vi "SoundMeasureWunan.vi"() -> ()   [LabVIEW 2016]
uses:
  <vilib>/Instr/_visa.llb/VISA Configure Serial Port (Instr).vi
  <vilib>/Utility/config.llb/Read Key (Double).vi
  <vilib>/Utility/file.llb/Write Delimited Spreadsheet (DBL).vi
  <vilib>/Utility/config.llb/NI_LVConfig.lvlib
panel:
  in  "record cycle":u64=7 min=6 step=1
  in  "freq (MHz)":dbl=1.36 min=0.1 max=10.0 step=0.01
  in  "SETVOLT":bool
  out "error out":errorcluster
  in  "cycle":u32=120
  in  "Channel":u16
  in  "KYCT axis in HIFU coordinate":cluster{"X axis":dbl[], "Z axis":dbl[]}={"X axis"=[1.0, 0.0, 0.0], "Z axis"=[0.0, 0.0, 1.0]}
  in  "KYCT coordinate":T1
  in  "Sens (V/MPa)":dbl=0.1284
  in  "Port":u32=12321
  in  "HIFU_connect":bool
  in  "HIFU_Telnet":bool
  out "Pressure (MPa)":dbl format="%#_4g"
  in  "pout":bool
  in  "totle chnnum":i16=64
  in  "HIFU IP":string="192.168.1.72"
  in  "SETPHS":bool
  out "XY Graph 2":T2(graph)
  in  "Set global voltage":bool
  in  "Voltage":dbl=4.0 min=0.5 max=20.0 step=1.0
  out "Sonication":bool
  in  "continuousOut":bool
  in  "Scan":bool
  in  "Tab Control":enum32{"1D Scan", "2D Scan", "Monitor"}(tab)
  out "1D plot":cluster{dbl[], dbl[]}(graph)
  out "2D Scan":dbl[][](graph)
  in  "start":bool
  in  "reord":bool
  out "Current":dbl[](graph)
  out "Voltage":dbl[](graph)
  in  "Go":bool
  in  "Speed":dbl=0.5 min=0.2 max=2.5 step=0.1
  in  "Position":dbl[](array[numeric]) step=5.0 format="%#_6f"
  in  "Z+":bool
  in  "Z-":bool
  in  "Y+":bool
  in  "Y-":bool
  in  "X+":bool
  in  "X-":bool
  in  "error in (no error)":errorcluster
  out "HIFU":bool
  out "osc":bool
  out "KYCT":bool
  in  "Exit":bool
  in  "3D motorized stage":refnum<visa-resource-name>
  in  "oscilloscope":refnum<visa-resource-name>
  # "Z"
  # "X"
  # "Y"
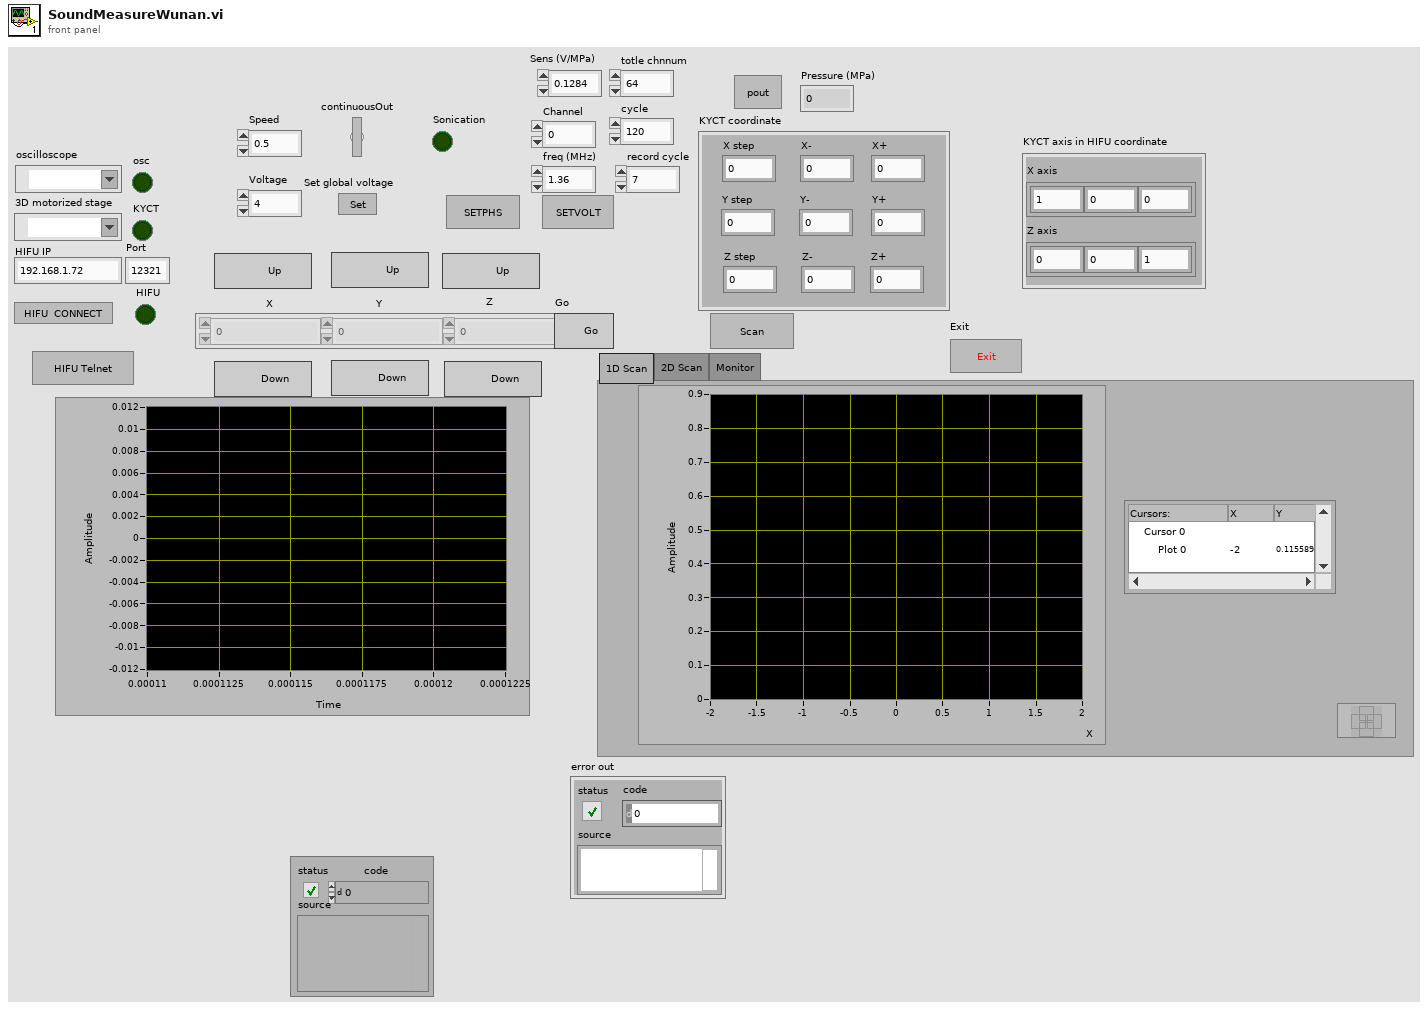
[diagram p1: front panel]
types:
  T1 = cluster{"X-":dbl, "X step":dbl, "Y-":dbl, "Y step":dbl, "Z-":dbl, "Z step":dbl, "Z+":dbl, "X+":dbl, "Y+":dbl}
  T2 = cluster{"time sequence":dbl[], "Voltage sequence":dbl[]}
  T3 = enum8{"Enabled", "Disabled", "Disabled and Grayed Out"}
  T4 = typedef "NI_LVConfig.lvlib/Config Data RefNum.ctl" = refnum<k1>
  T5 = typedef "NI_Matrix.lvlib/RealMatrix.ctl" = dbl[][]
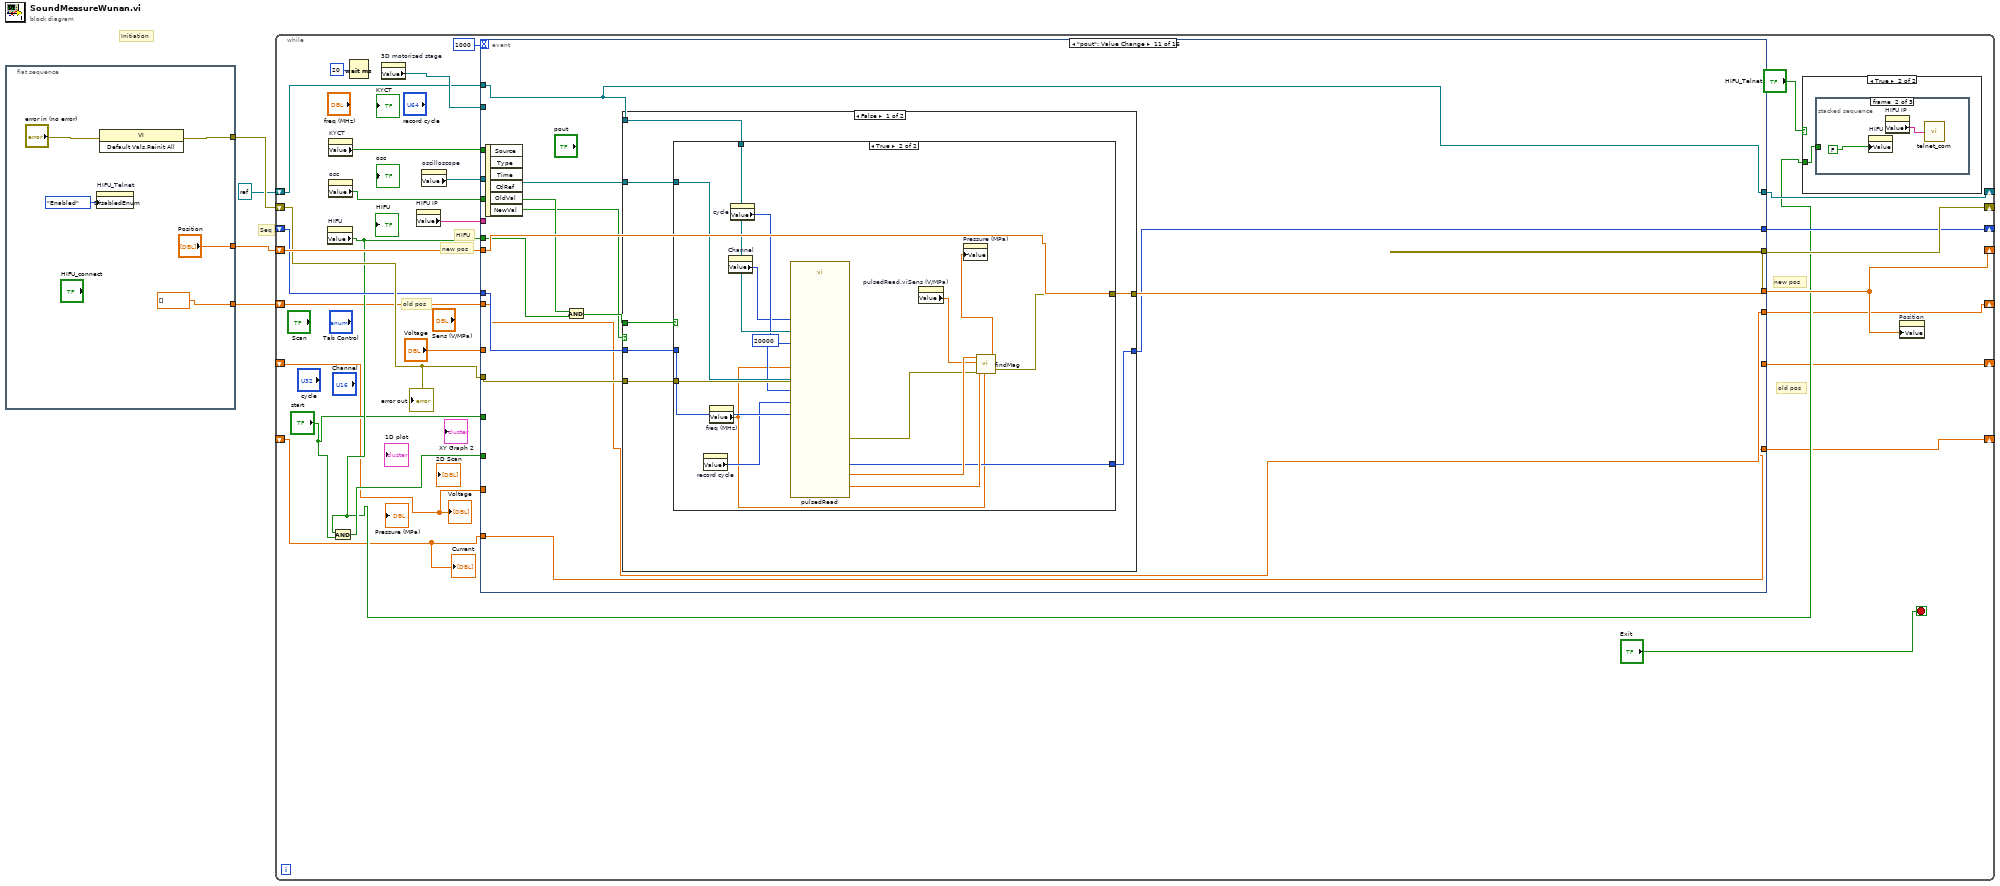
[diagram p0: block diagram]
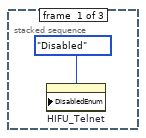
[diagram p3: hidden frame]
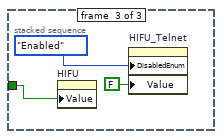
[diagram p4: hidden frame]
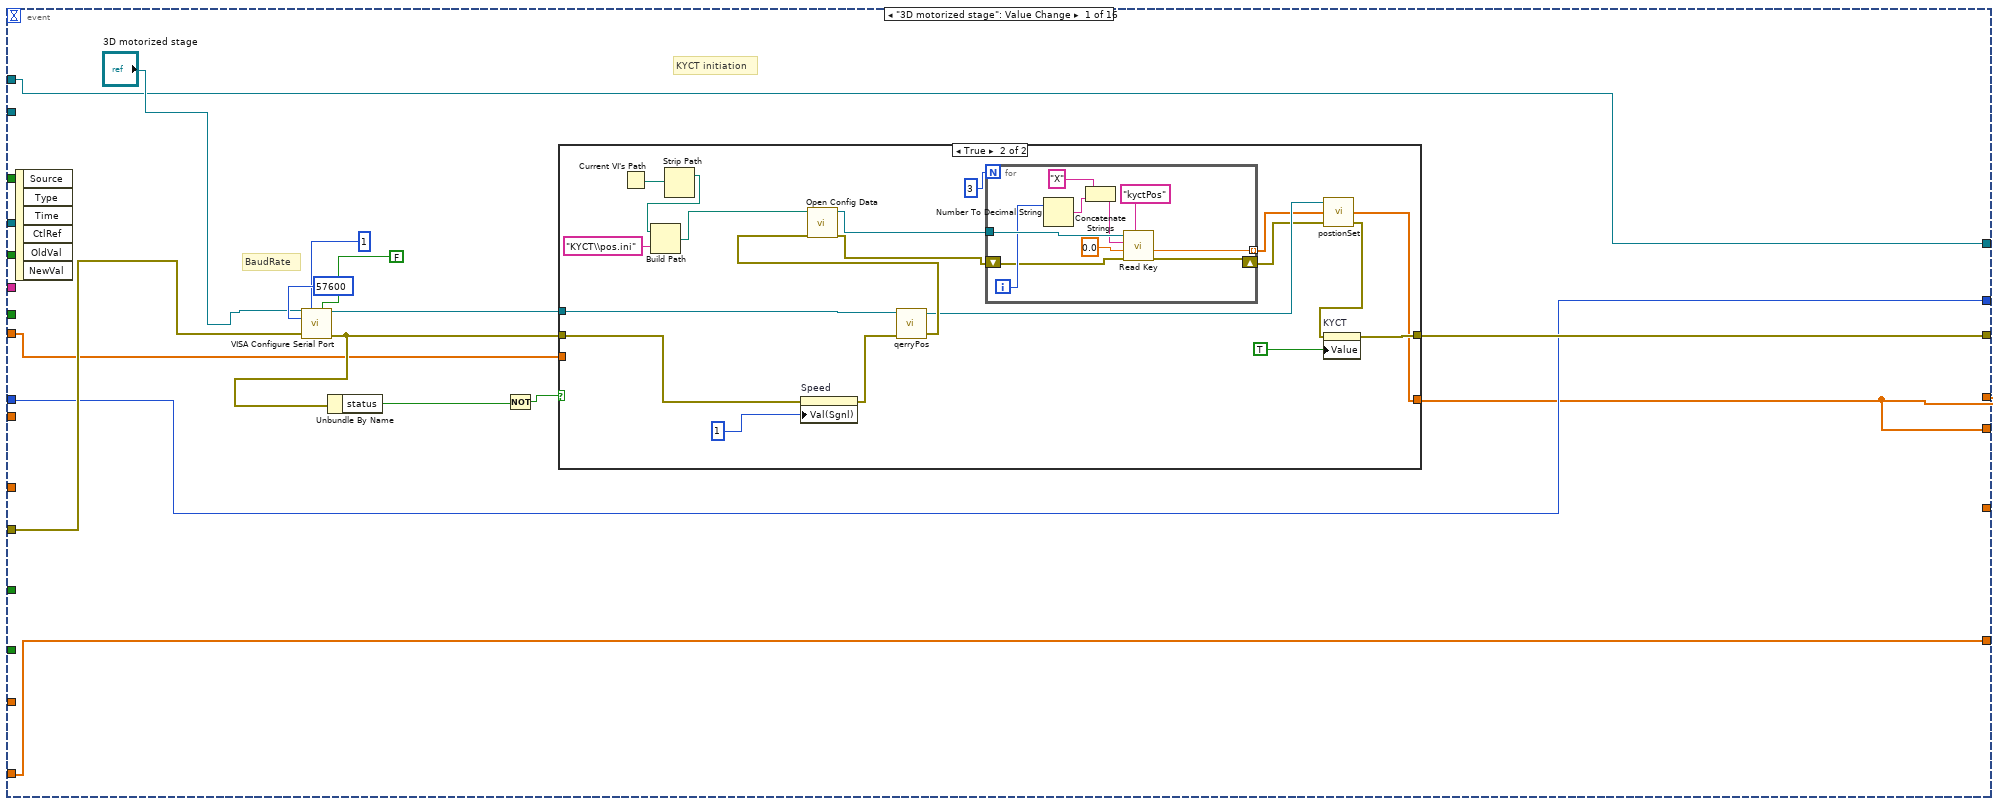
[diagram p5: hidden frame]
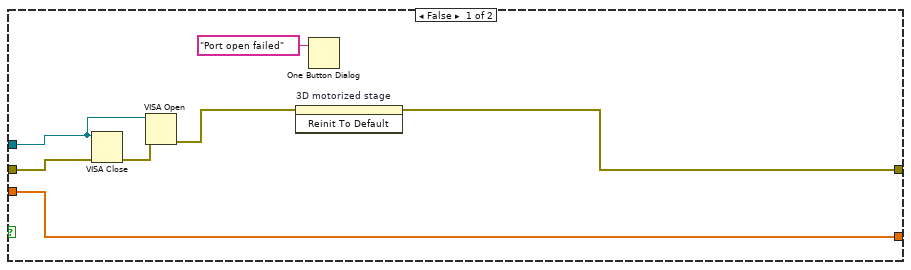
[diagram p6: hidden frame]
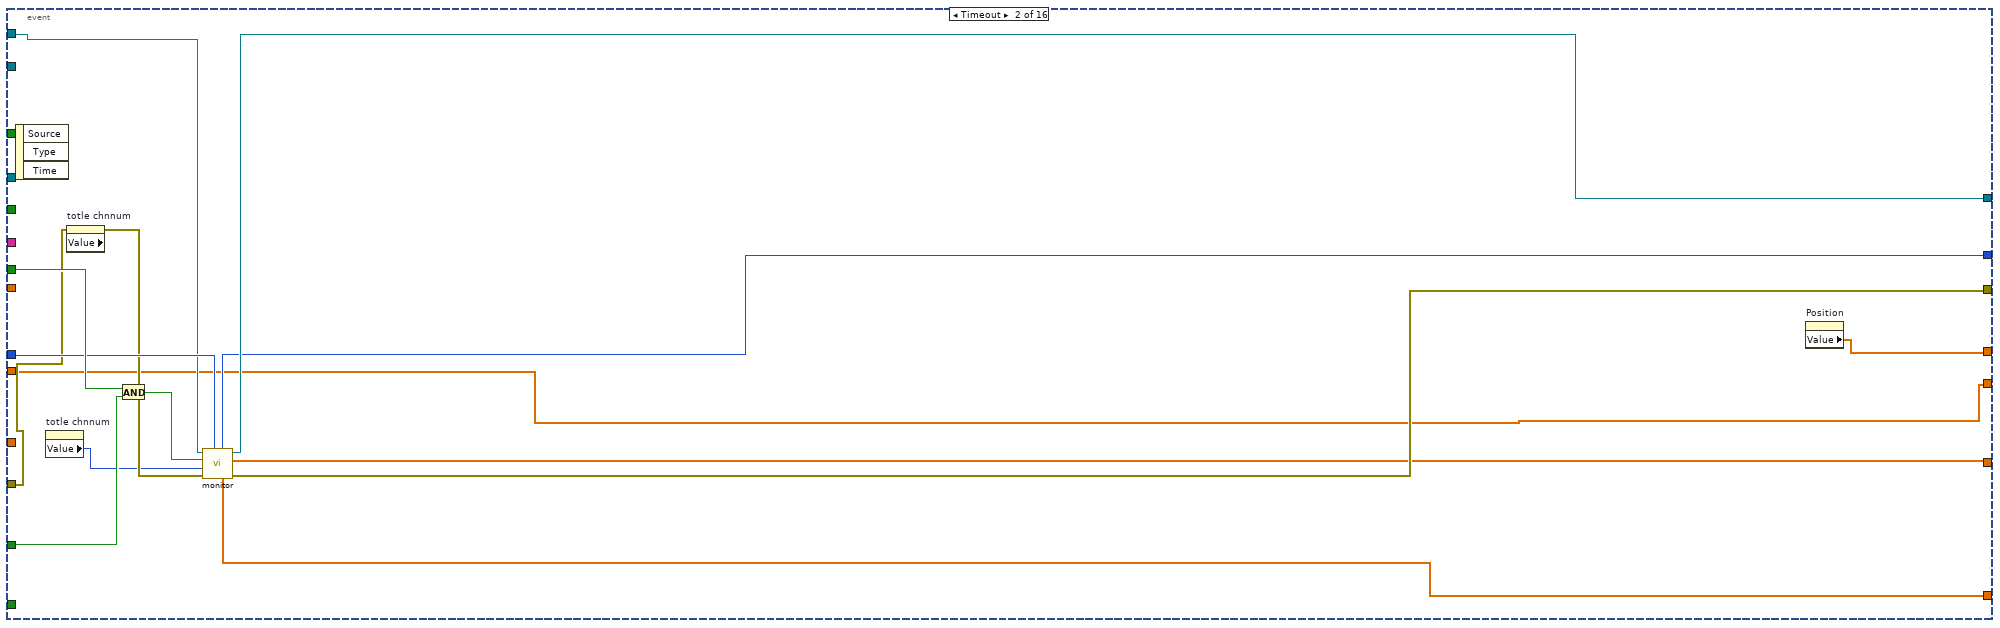
[diagram p7: hidden frame]
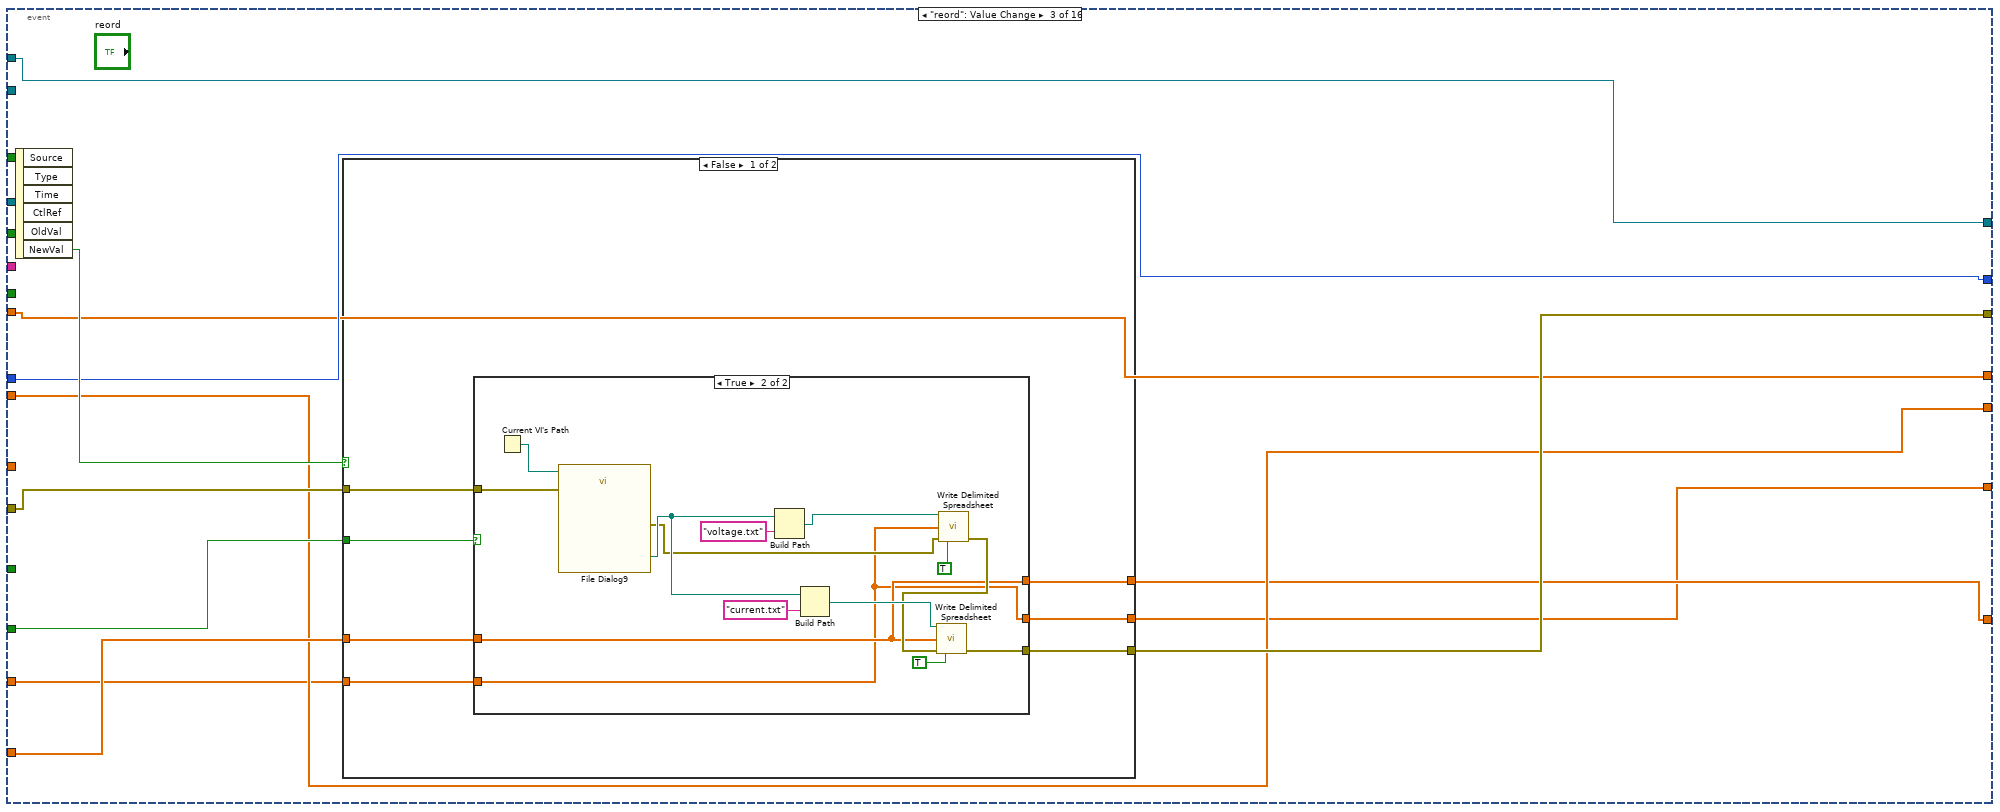
[diagram p8: hidden frame]
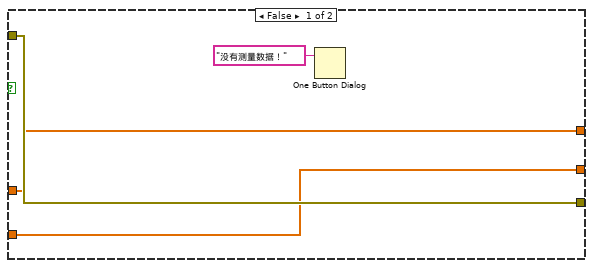
[diagram p9: hidden frame]
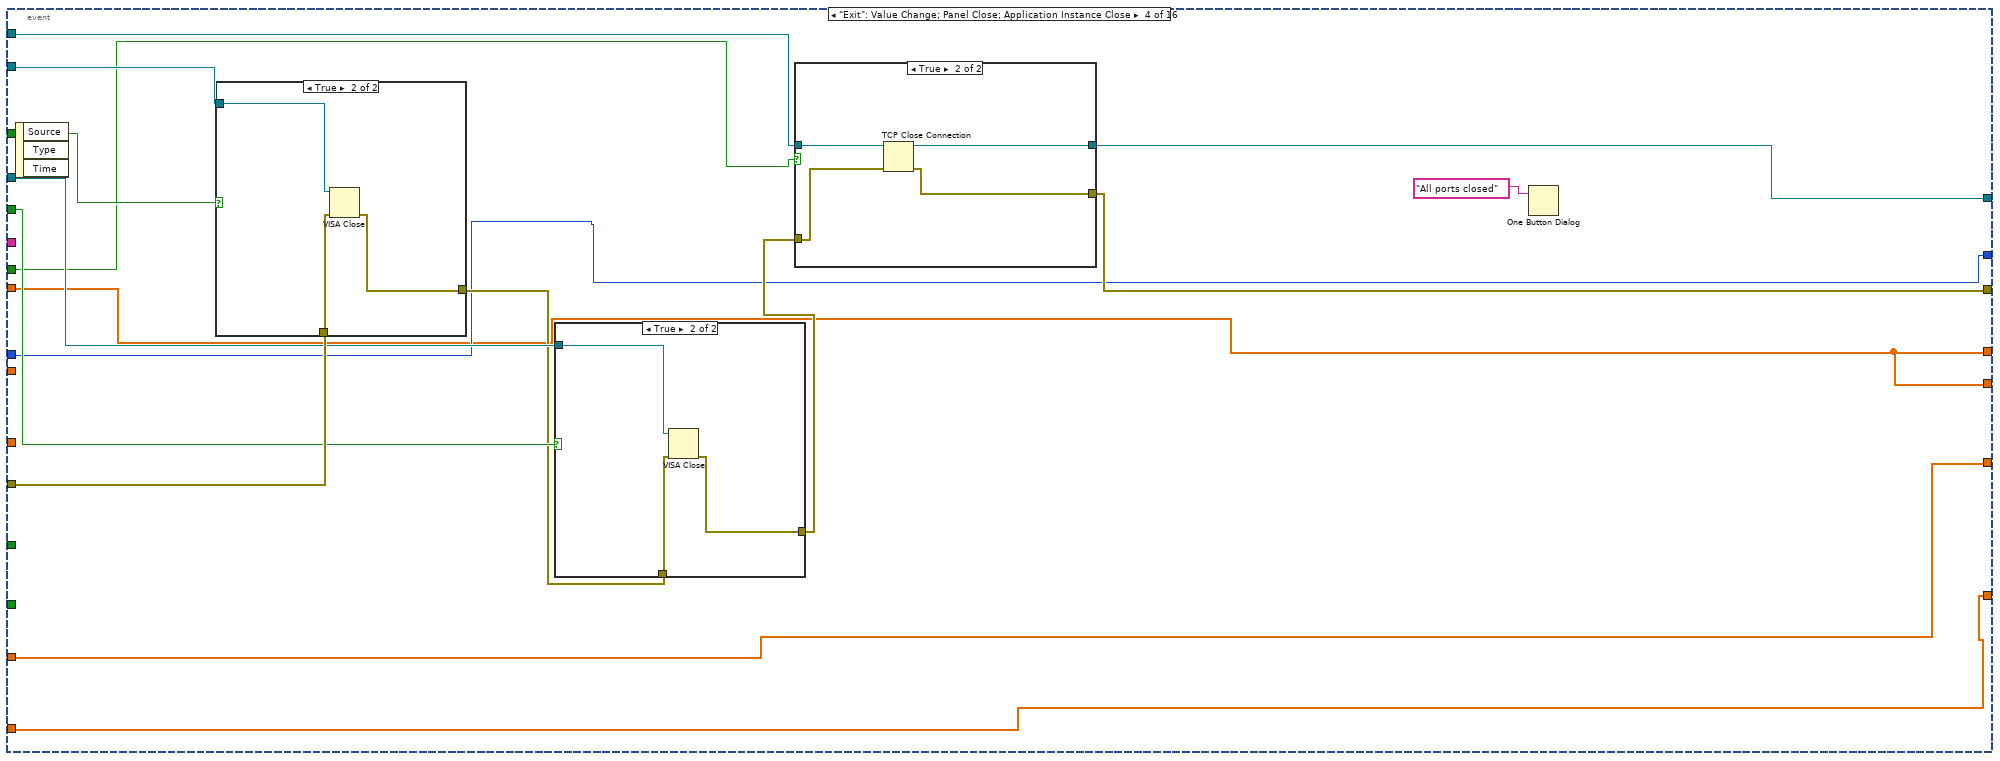
[diagram p11: hidden frame]
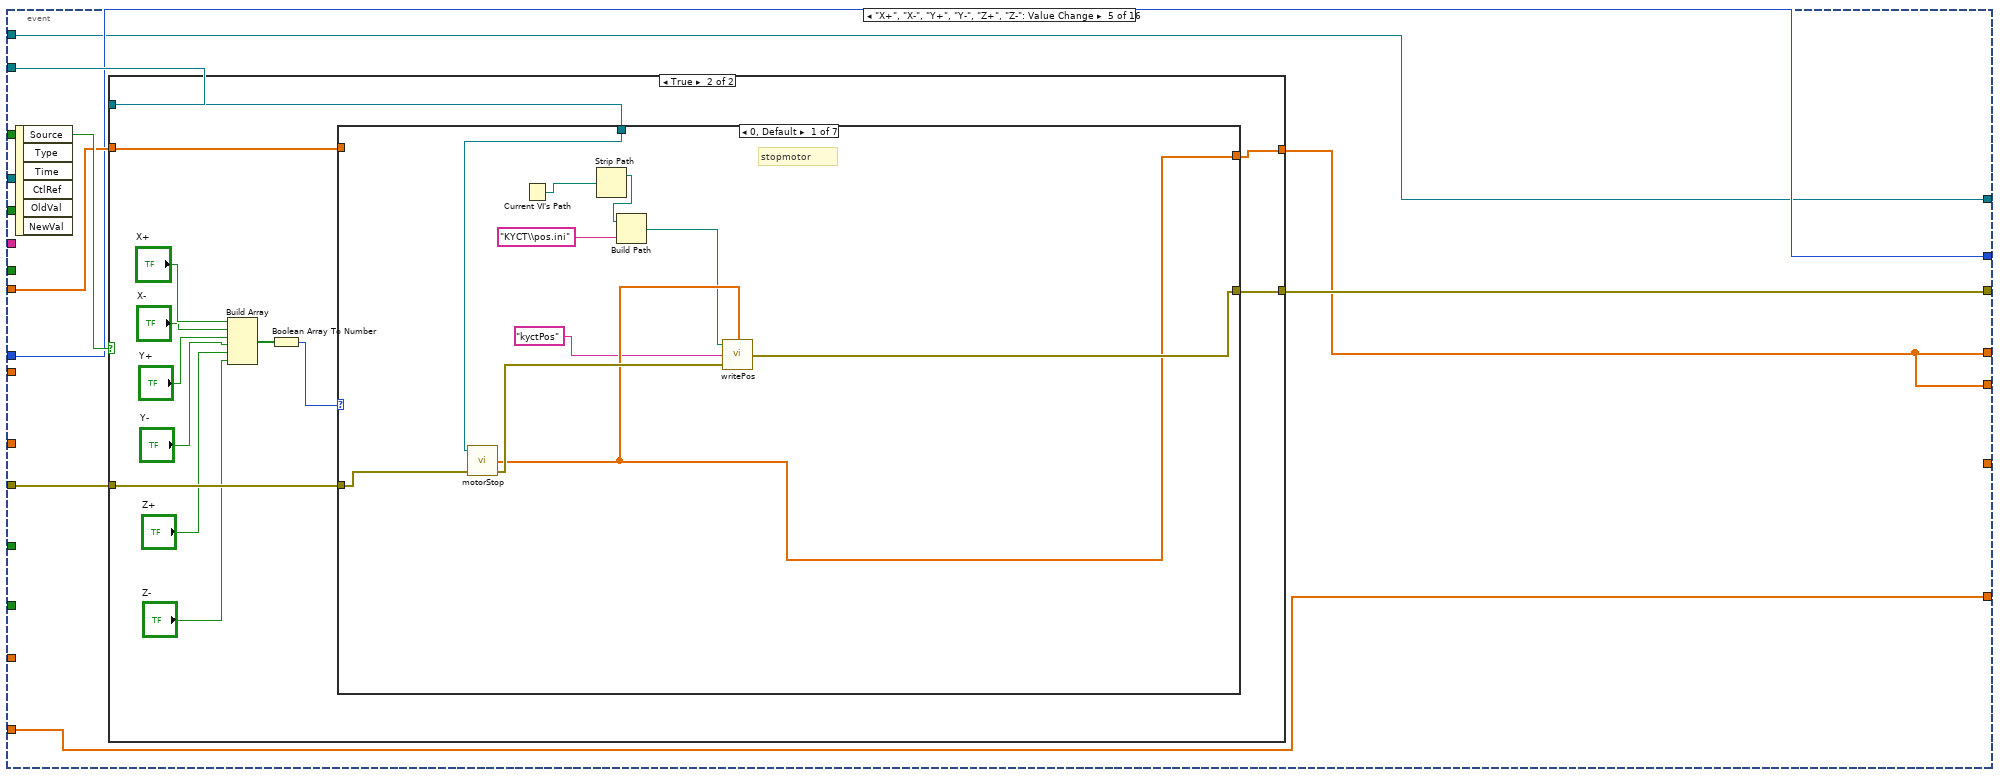
[diagram p15: hidden frame]
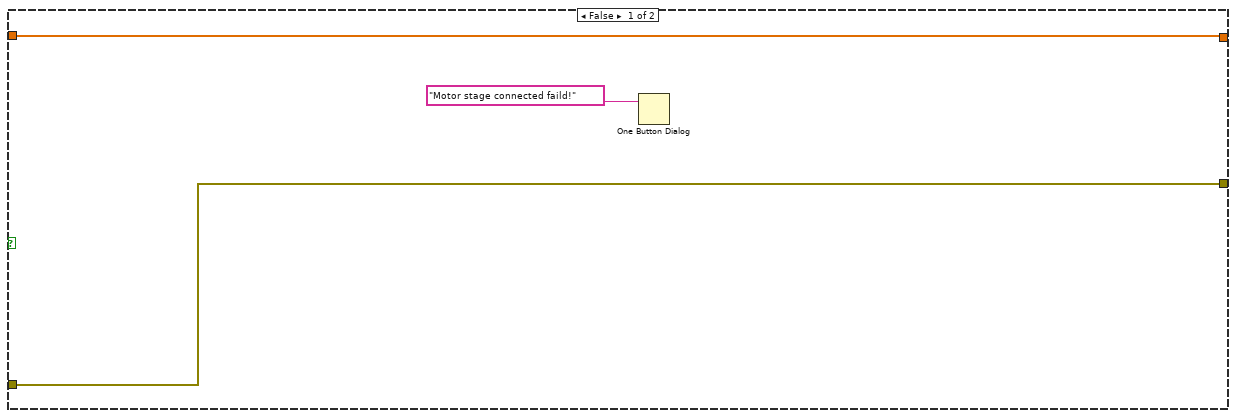
[diagram p16: hidden frame]
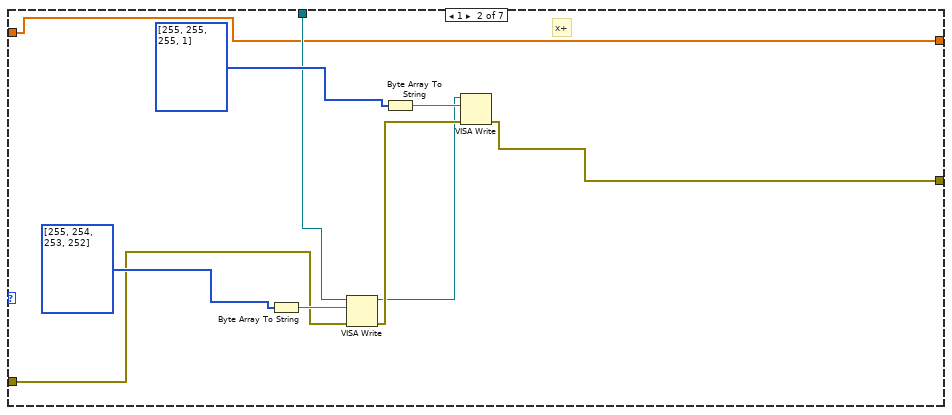
[diagram p17: hidden frame]
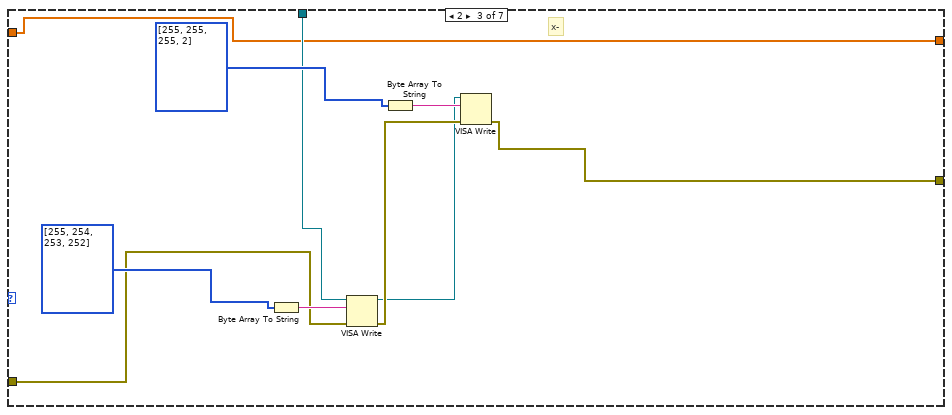
[diagram p18: hidden frame]
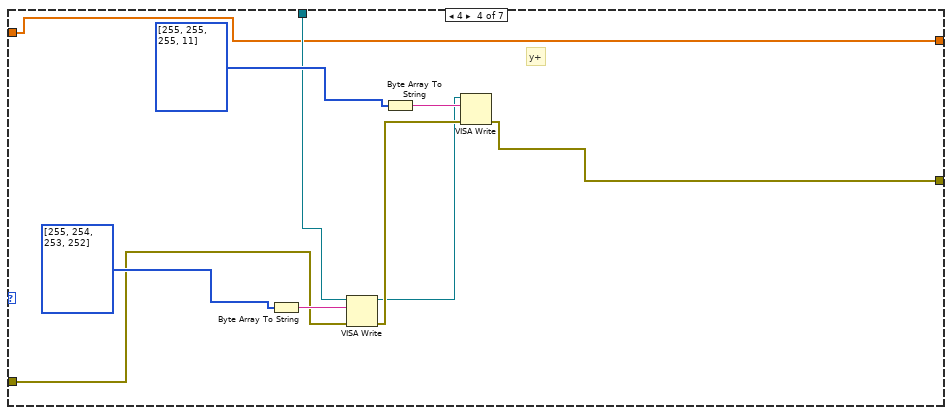
[diagram p19: hidden frame]
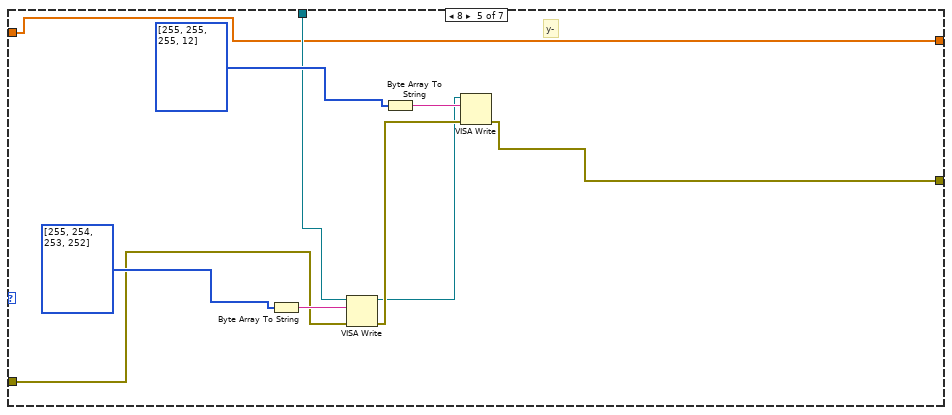
[diagram p20: hidden frame]
diagram:
  # "Seq"
  # "Initiation"
  n1 = flat-sequence {
    tunnel: ["Position"] -> w4
    tunnel: [w8] -> w3
    tunnel: [dbl[] []] -> w1
    frame #0 {
      n2 = property on="HIFU_Telnet" class="Bool (strict)"("DisabledEnum"=T3."Enabled" ("Disabled")) -> ()  [unwired: 2 in, 2 out]
      n3 = invoke class="VI" method="Default Vals.Reinit All"(error in="error in (no error)") -> (error out=w8:errorcluster)  [unwired: 2 in, 2 out]
    }
  }
  n4 = while {
    shift-right: [w34] -> _
    shift-left: w4 -> [w33]
    shift-right: [w32] -> _
    shift-left: w3 -> [w20]
    shift-right: [w23] -> _
    shift-left: refnum<k5> refnum ("connection ID out") -> [w22]
    shift-right: [w21] -> _
    shift-left: _ -> [w19]
    shift-right: [w17] -> _
    shift-left: _ -> [w16]
    shift-right: [w13] -> _
    shift-left: w1 -> [w12]
    shift-right: [w11] -> _
    shift-left: _ -> [w10]
    stop <- "Exit" stop-if-true
    # "HIFU"
    # "old pos"
    # "new pos"
    # "old pos"
    # "new pos"
    n5 = property on="HIFU" class="Bool (strict)"() -> ("Value"=w18:bool)  [unwired: 2 in, 2 out]
    n6 = property on="KYCT" class="Bool (strict)"() -> ("Value"=w36:bool)  [unwired: 2 in, 2 out]
    n7 = property on="osc" class="Bool (strict)"() -> ("Value"=w35:bool)  [unwired: 2 in, 2 out]
    n8 = And(x=w18, y="start") -> (x .and. y?=w25:bool)
    n9 = Wait (ms)(milliseconds to wait=u32 20) -> ()  [unwired: 1 out]
    n10 = property on="3D motorized stage" class="VISAName"() -> ("Value"=w30:refnum<visa-resource-name>)  [unwired: 2 in, 2 out]
    n11 = property on="HIFU IP" class="Str"() -> ("Value"=w26:string)  [unwired: 2 in, 2 out]
    n12 = property on="oscilloscope" class="VISAName"() -> ("Value"=w29:refnum<visa-resource-name>)  [unwired: 2 in, 2 out]
    n13 = event shown="[10] \"pout\": Value Change" {
      selector: _ -> [_ _ _ _ _ _ _ _ _ _ _ _ _ _ _ _]
      dyn-events: _ -> [_ _ _ _ _ _ _ _ _ _ _ _ _ _ _ _]
      timeout: 1000 -> [_ _ _ _ _ _ _ _ _ _ _ _ _ _ _ _]
      tunnel: w30 -> [_ _ _ w164 w187 w283 w304 _ _ w423 _ _ _ _ _ _]
      tunnel: w29 -> [_ _ _ w161 _ _ _ _ _ w421 w659 _ _ _ _ _]
      tunnel: w20 -> [w54 w107 w121 w163 w186 w284 w303 w335 w377 w422 w658 w699 w709 w745 w760 w792]
      tunnel: w36 -> [_ _ _ w165 w188 w282 w305 _ _ w428 _ _ _ _ _ w796]
      tunnel: [w56 w99 w119 w155 w185 w280 w301 w333 w375 w420 w657 w698 w707 w745 w759 w791] -> w32
      tunnel: w35 -> [_ _ _ w162 _ _ _ _ _ w427 w656 _ _ _ _ _]
      tunnel: w33 -> [w49 _ w114 w152 w184 w277 _ w336 w378 w419 w660 w700 w710 w747 w757 w795]
      tunnel: [w45 w97 w114 w152 w181 w277 w296 w336 w378 w413 w660 w700 w710 w747 w757 w794] -> w34
      tunnel: w18 -> [_ w109 _ w158 _ _ _ w334 w376 w426 w655 _ _ _ w756 w789]
      tunnel: "Voltage" -> [_ _ _ _ _ _ _ _ _ _ _ _ _ _ w758 _]
      tunnel: w16 -> [w44 _ w120 w150 w180 w275 w293 w327 w369 w411 w648 w693 w702 w749 w750 w782]
      tunnel: w26 -> [_ _ _ _ _ _ _ _ _ w418 _ _ _ _ _ w788]
      tunnel: w25 -> [_ _ w118 _ _ _ _ _ _ _ _ _ _ _ _ _]
      tunnel: [w47 w103 w116 w153 w182 w278 w298 w331 w373 w414 w650 w695 w705 w743 w752 w784] -> w23
      tunnel: w22 -> [w47 w104 w116 w156 w182 w278 w298 w331 w373 w414 w650 w695 _ w743 w752 w787]
      tunnel: [w46 w101 w115 w154 w183 w279 w299 w329 w371 w415 w651 w696 w704 w744 w753 w785] -> w21
      tunnel: w19 -> [w46 w108 w115 w154 w183 w279 w299 w330 w372 w416 w652 w696 _ w744 w754 w786]
      tunnel: [w44 w102 w111 w150 w180 w275 w293 w327 w369 w411 w648 w693 w702 w749 w750 w782] -> w17
      tunnel: "start" -> [_ w100 _ _ _ _ _ _ _ _ _ _ _ _ _ _]
      tunnel: [w45 w96 w113 w152 w181 w276 w295 w328 w370 w413 w649 w694 w703 w746 w751 w783] -> w13
      tunnel: w12 -> [_ w96 w113 _ _ w276 w297 w328 w370 w412 w649 w694 w703 w746 w751 w783]
      tunnel: [_ w95 w110 w151 _ _ _ _ _ _ _ _ _ w748 _ w781] -> w11
      tunnel: w10 -> [_ _ w112 w151 _ _ _ _ _ _ _ _ _ w748 _ w781]
      event "3D motorized stage": Value Change {
        # "KYCT initiation"
        # "BaudRate"
        n14 = event-data() -> ()  [unwired: 1 in, 6 out]
        n15 = call-poly "VISA Configure Serial Port"("VISA resource name"="3D motorized stage", "timeout (10sec)"=u32 1, "Enable Termination\nChar (T)"=FALSE, "baud rate (9600)"=u32 57600, "error in (no error)"=w54) -> ("VISA resource name out"=w57:refnum<visa-resource-name>, "error out"=w52:errorcluster)  [unwired: 9 in]
        n16 = Unbundle By Name(w52) -> ("status"=w51:bool)
        n17 = Not(x=w51) -> (.not. x?=w50:bool)
        n18 = case shown="True" w50 {
          tunnel: w57 -> [w59 w82]
          tunnel: [w65 w67] -> w45
          tunnel: [w64 w81] -> w56
          tunnel: w52 -> [w62 w79]
          tunnel: w49 -> [w65 _]
          frame False {
            n19 = VISA Close(VISA resource name=w59, error in (no error)=w62) -> (error out=w61:errorcluster)
            n20 = VISA Open(error in (no error)=w61, VISA resource name=w59) -> (error out=w60:errorcluster)  [unwired: 3 in, 1 out]
            n21 = invoke on="3D motorized stage" class="VISAName" method="Reinit To Default"(error in=w60) -> (error out=w64:errorcluster)  [unwired: 2 in, 2 out]
            n22 = One Button Dialog(message="Port open failed") -> ()  [unwired: 1 in, 1 out]
          }
          frame True {
            n23 = Current VI's Path() -> (path=w78:path)
            n24 = Strip Path(path=w78) -> (stripped path=w77:path)  [unwired: 1 out]
            n25 = Build Path(base path=w77, name or relative path="KYCT\\pos.ini") -> (appended path=w75:path)
            n26 = property on="Speed" class="DigNum (strict)"(error in=w79, "Val(Sgnl)"=1) -> (error out=w80:errorcluster)  [unwired: 1 in, 1 out]
            n27 = call "qerryPos.vi"("error in (no error)"=w80, "UART in"=w82) -> ("error out"=w74:errorcluster, "UART out"=w70:refnum<visa-resource-name>)  [unwired: 2 in, 1 out]
            n28 = call <vilib>:"Open Config Data.vi"("error in (no error)"=w74, "configuration file path"=w75) -> ("error out"=w72:errorcluster, "refnum"=w71:T4)  [unwired: 7 in, 1 out]
            n29 = for {
              N: 3 -> [_]
              tunnel: w71 -> [w94]
              shift-right: [w87] -> w69
              shift-left: w72 -> [w88]
              tunnel: [w86] -> w68 mode=indexing
              i -> [w90]
              n30 = Number To Decimal String(number=w90) -> (decimal integer string=w92:string)  [unwired: 1 in]
              n31 = Concatenate Strings("X" ("string"), w92) -> (w91:string)
              n32 = call-poly <vilib>:"Read Key.vi"("section"="kyctPos", "error in (no error)"=w88, "default value"=0.0, "key"=w91, "refnum"=w94) -> ("error out"=w87:errorcluster, "value"=w86:dbl)  [unwired: 3 in, 2 out]
            }
            n33 = call "postionSet.vi"("error in (no error)"=w69, "Pos in"=w68, "UART PORT in"=w70) -> ("error out"=w66:errorcluster, "Pos out"=w67:dbl[])  [unwired: 1 out]
            n34 = property on="KYCT" class="Bool (strict)"(error in=w66, "Value"=TRUE) -> (error out=w81:errorcluster)  [unwired: 1 in, 1 out]
          }
        }
      }
      event Timeout {
        n35 = event-data() -> ()  [unwired: 1 in, 3 out]
        n36 = property on="totle chnnum" class="DigNum (strict)"() -> ("Value"=w98:i16)  [unwired: 2 in, 2 out]
        n37 = property on="totle chnnum" class="DigNum (strict)" props=["Value"](error in=w107) -> (error out=w106:errorcluster)  [unwired: 1 in, 2 out]
        n38 = And(x=w109, y=w100) -> (x .and. y?=w105:bool)
        n39 = call "monitor.vi"("HIFU_TCP in"=w104, "HIFU"=w105, "chn num"=w98, "error in (no error)"=w106, "sequence"=w108) -> ("SEQ out"=w101:u32, "current"=w102:dbl[], "HIFU_TCP out"=w103:refnum<k5>, "voltage"=w95:dbl[], "error out"=w99:errorcluster)  [unwired: 1 out]
        n40 = property on="Position" class="Arr (strict)"() -> ("Value"=w97:dbl[])  [unwired: 2 in, 2 out]
      }
      event "reord": Value Change {
        n41 = event-data() -> ("NewVal"=w117:bool)  [unwired: 1 in, 5 out]
        n42 = case shown="False" w117 {
          tunnel: w121 -> [w128 w149]
          tunnel: w120 -> [w127 w148]
          tunnel: [w126 w149] -> w119
          tunnel: w118 -> [w125 _]
          tunnel: w112 -> [w124 w147]
          tunnel: [w123 w148] -> w111
          tunnel: [w122 w147] -> w110
          frame False {
            n43 = case shown="True" w125 {
              tunnel: w128 -> [w132 w141]
              tunnel: w127 -> [w130 w134]
              tunnel: [w132 w137] -> w126
              tunnel: w124 -> [w129 w133]
              tunnel: [w130 w134] -> w123
              tunnel: [w129 w133] -> w122
              frame False {
                n44 = One Button Dialog(message="没有测量数据！") -> ()  [unwired: 1 in, 1 out]
              }
              frame True {
                n45 = Current VI's Path() -> (path=w146:path)
                n46 = call "File Dialog9"("start path"=w146, "error in"=w141) -> ("selected path"=w143:path, "error out"=w140:errorcluster)  [unwired: 10 in, 2 out]
                n47 = Build Path(base path=w143, name or relative path="voltage.txt") -> (appended path=w142:path)
                n48 = Build Path(base path=w143, name or relative path="current.txt") -> (appended path=w139:path)
                n49 = call-poly <vilib>:"Write Delimited Spreadsheet.vi"("file path (dialog if empty)"=w142, "1D data"=w133, "error in (no error)"=w140, "transpose? (no:F)"=TRUE) -> ("error out"=w138:errorcluster)  [unwired: 10 in, 1 out]
                n50 = call-poly <vilib>:"Write Delimited Spreadsheet.vi"("file path (dialog if empty)"=w139, "1D data"=w134, "error in (no error)"=w138, "transpose? (no:F)"=TRUE) -> ("error out"=w137:errorcluster)  [unwired: 10 in, 1 out]
              }
            }
          }
          frame True {
          }
        }
      }
      event "Exit": Value Change; Panel Close; Application Instance Close {
        n51 = event-data() -> ()  [unwired: 1 in, 3 out]
        n52 = case shown="True" w165 {
          tunnel: w164 -> [_ w179]
          tunnel: w163 -> [w176 w178]
          tunnel: [w176 w177] -> w160
          frame False {
          }
          frame True {
            n53 = VISA Close(VISA resource name=w179, error in (no error)=w178) -> (error out=w177:errorcluster)
          }
        }
        n54 = case shown="True" w162 {
          tunnel: w161 -> [_ w175]
          tunnel: w160 -> [w172 w174]
          tunnel: [w172 w173] -> w157
          frame False {
          }
          frame True {
            n55 = VISA Close(VISA resource name=w175, error in (no error)=w174) -> (error out=w173:errorcluster)
          }
        }
        n56 = case shown="True" w158 {
          tunnel: w157 -> [w167 w170]
          tunnel: w156 -> [w166 w171]
          tunnel: [w167 w169] -> w155
          tunnel: [w166 w168] -> w153
          frame False {
          }
          frame True {
            n57 = TCP Close Connection(connection ID=w171, error in (no error)=w170) -> (connection ID out=w168:refnum<k5>, error out=w169:errorcluster)  [unwired: 1 in]
          }
        }
        n58 = One Button Dialog(message="All ports closed") -> ()  [unwired: 1 in, 1 out]
      }
      event "X+", "X-", "Y+", "Y-", "Z+", "Z-": Value Change {
        n59 = event-data() -> ()  [unwired: 1 in, 6 out]
        n60 = case shown="True" w188 {
          tunnel: w187 -> [_ w203]
          tunnel: w186 -> [w190 w204]
          tunnel: [w190 w202] -> w185
          tunnel: [w189 w200] -> w181
          tunnel: w184 -> [w189 w201]
          frame False {
            n61 = One Button Dialog(message="Motor stage connected faild!") -> ()  [unwired: 1 in, 1 out]
          }
          frame True {
            n62 = Build Array("X+", "X-", "Y+", "Y-", "Z+", "Z-") -> (w193:bool[])
            n63 = Boolean Array To Number(Boolean array=w193) -> (number=w192:u32)
            n64 = case shown="0, Default" w192 {
              tunnel: w204 -> [w214 w220 w230 w240 w250 w260 w270]
              tunnel: w203 -> [w213 w219 w229 w239 w249 w259 w269]
              tunnel: [w211 w216 w226 w236 w246 w256 w266] -> w202
              tunnel: w201 -> [_ w215 w225 w235 w245 w255 w265]
              tunnel: [w210 w215 w225 w235 w245 w255 w265] -> w200
              frame 0, Default {
                # "stopmotor"
                n65 = call "motorStop.vi"("error in (no error)"=w214, "UART PORT in"=w213) -> ("error out"=w212:errorcluster, "P1"=w210:dbl[])  [unwired: 1 in, 1 out]
                n66 = Current VI's Path() -> (path=w208:path)
                n67 = Strip Path(path=w208) -> (stripped path=w207:path)  [unwired: 1 out]
                n68 = Build Path(base path=w207, name or relative path="KYCT\\pos.ini") -> (appended path=w206:path)
                n69 = call "writePos.vi"("Pos"=w210, "error in (no error)"=w212, "name"="kyctPos", "ini Path in"=w206) -> ("error out"=w211:errorcluster)
              }
              frame 1 {
                # "x+"
                n70 = Byte Array To String(unsigned byte array=i32[] [255, 254, 253, 252]) -> (string=w222:string)
                n71 = VISA Write(VISA resource name=w219, write buffer=w222, error in (no error)=w220) -> (VISA resource name out=w217:refnum<visa-resource-name>, error out=w218:errorcluster)  [unwired: 1 out]
                n72 = Byte Array To String(unsigned byte array=i32[] [255, 255, 255, 1]) -> (string=w224:string)
                n73 = VISA Write(VISA resource name=w217, write buffer=w224, error in (no error)=w218) -> (error out=w216:errorcluster)  [unwired: 2 out]
              }
              frame 2 {
                # "x-"
                n74 = Byte Array To String(unsigned byte array=i32[] [255, 254, 253, 252]) -> (string=w232:string)
                n75 = VISA Write(VISA resource name=w229, write buffer=w232, error in (no error)=w230) -> (VISA resource name out=w227:refnum<visa-resource-name>, error out=w228:errorcluster)  [unwired: 1 out]
                n76 = Byte Array To String(unsigned byte array=i32[] [255, 255, 255, 2]) -> (string=w234:string)
                n77 = VISA Write(VISA resource name=w227, write buffer=w234, error in (no error)=w228) -> (error out=w226:errorcluster)  [unwired: 2 out]
              }
              frame 4 {
                # "y+"
                n78 = Byte Array To String(unsigned byte array=i32[] [255, 254, 253, 252]) -> (string=w242:string)
                n79 = VISA Write(VISA resource name=w239, write buffer=w242, error in (no error)=w240) -> (VISA resource name out=w237:refnum<visa-resource-name>, error out=w238:errorcluster)  [unwired: 1 out]
                n80 = Byte Array To String(unsigned byte array=i32[] [255, 255, 255, 11]) -> (string=w244:string)
                n81 = VISA Write(VISA resource name=w237, write buffer=w244, error in (no error)=w238) -> (error out=w236:errorcluster)  [unwired: 2 out]
              }
              frame 8 {
                # "y-"
                n82 = Byte Array To String(unsigned byte array=i32[] [255, 254, 253, 252]) -> (string=w252:string)
                n83 = VISA Write(VISA resource name=w249, write buffer=w252, error in (no error)=w250) -> (VISA resource name out=w247:refnum<visa-resource-name>, error out=w248:errorcluster)  [unwired: 1 out]
                n84 = Byte Array To String(unsigned byte array=i32[] [255, 255, 255, 12]) -> (string=w254:string)
                n85 = VISA Write(VISA resource name=w247, write buffer=w254, error in (no error)=w248) -> (error out=w246:errorcluster)  [unwired: 2 out]
              }
              frame 16 {
                # "z+"
                n86 = Byte Array To String(unsigned byte array=i32[] [255, 254, 253, 252]) -> (string=w262:string)
                n87 = VISA Write(VISA resource name=w259, write buffer=w262, error in (no error)=w260) -> (VISA resource name out=w257:refnum<visa-resource-name>, error out=w258:errorcluster)  [unwired: 1 out]
                n88 = Byte Array To String(unsigned byte array=i32[] [255, 255, 255, 21]) -> (string=w264:string)
                n89 = VISA Write(VISA resource name=w257, write buffer=w264, error in (no error)=w258) -> (error out=w256:errorcluster)  [unwired: 2 out]
              }
              frame 32 {
                # "z-"
                n90 = Byte Array To String(unsigned byte array=i32[] [255, 254, 253, 252]) -> (string=w272:string)
                n91 = VISA Write(VISA resource name=w269, write buffer=w272, error in (no error)=w270) -> (VISA resource name out=w267:refnum<visa-resource-name>, error out=w268:errorcluster)  [unwired: 1 out]
                n92 = Byte Array To String(unsigned byte array=i32[] [255, 255, 255, 22]) -> (string=w274:string)
                n93 = VISA Write(VISA resource name=w267, write buffer=w274, error in (no error)=w268) -> (error out=w266:errorcluster)  [unwired: 2 out]
              }
            }
          }
        }
      }
      event "Speed": Value Change {
        n94 = event-data() -> ()  [unwired: 1 in, 6 out]
        n95 = case shown="False" w282 {
          tunnel: "Speed" -> [_ w292]
          tunnel: w284 -> [w286 w291]
          tunnel: w283 -> [_ w290]
          tunnel: [w286 w287] -> w280
          frame False {
            n96 = One Button Dialog(message="Motor stage connected faild!") -> ()  [unwired: 1 in, 1 out]
          }
          frame True {
            n97 = call "setVel.vi"("error in (no error)"=w291, "speed"=w292, "UART in"=w290) -> ("error out"=w289:errorcluster, "UART out"=w288:refnum<visa-resource-name>)
            n98 = property on="3D motorized stage" class="VISAName"(error in=w289, "Value"=w288) -> (error out=w287:errorcluster)  [unwired: 1 in, 1 out]
          }
        }
      }
      event "Go": Value Change {
        n99 = event-data() -> ("NewVal"=w300:bool)  [unwired: 1 in, 5 out]
        n100 = property on="Position" class="Arr (strict)"() -> ("Value"=w294:dbl[])  [unwired: 2 in, 2 out]
        n101 = case shown="True" w305 {
          tunnel: w304 -> [_ w317]
          tunnel: w303 -> [w308 w316]
          tunnel: [w307 w312] -> w296
          tunnel: [w308 w315] -> w302
          tunnel: w294 -> [w307 w313]
          tunnel: w300 -> [_ w314]
          tunnel: w297 -> [w306 w311]
          tunnel: [w306 w310] -> w295
          frame False {
            n102 = One Button Dialog(message="Motor stage connected faild!") -> ()  [unwired: 1 in, 1 out]
          }
          frame True {
            n103 = case shown="False" w314 {
              tunnel: w317 -> [w323 _]
              tunnel: w316 -> [w322 w326]
              tunnel: [w321 w326] -> w315
              tunnel: [w318 w325] -> w312
              tunnel: w313 -> [w320 w325]
              tunnel: w311 -> [w319 w324]
              tunnel: [w318 w324] -> w310
              frame False {
                n104 = call "move.vi"("error in (no error)"=w322, "P01"=w320, "P0"=w319, "UART PORT in"=w323) -> ("error out"=w321:errorcluster, "P1"=w318:dbl[])  [unwired: 1 out]
              }
              frame True {
              }
            }
          }
        }
        n105 = invoke on="Go" class="Bool" method="Reinit To Default"(error in=w302) -> (error out=w301:errorcluster)  [unwired: 2 in, 2 out]
      }
      event "SETPHS": Value Change {
        n106 = event-data() -> ("NewVal"=w332:bool)  [unwired: 1 in, 5 out]
        n107 = case shown="True" w334 {
          tunnel: w335 -> [w339 w344]
          tunnel: [w339 w345] -> w333
          tunnel: w332 -> [_ w343]
          tunnel: w331 -> [_ w342]
          tunnel: w330 -> [w337 w341]
          tunnel: [w337 w340] -> w329
          frame False {
            n108 = One Button Dialog(message="i2c connected failed") -> ()  [unwired: 1 in, 1 out]
          }
          frame True {
            n109 = case shown="False" w343 {
              tunnel: [w353 w368] -> w345
              tunnel: w344 -> [w352 w368]
              tunnel: w342 -> [w349 _]
              tunnel: w341 -> [w347 w367]
              tunnel: [w346 w367] -> w340
              frame False {
                n110 = call "File Dialog8"("error in"=w352) -> ("selected path"=w356:path, "error out"=w351:errorcluster)  [unwired: 11 in, 2 out]
                n111 = case shown="No Error" w351 {
                  selector: w351 -> [w357 w363]
                  tunnel: w356 -> [w360 _]
                  tunnel: [w359 w364] -> w355
                  tunnel: [w358 w362] -> w354
                  frame No Error {
                    n112 = call "readPHS.vi"("error in (no error)"=w357, "Path"=w360) -> ("error out"=w358:errorcluster, "Array"=w359:sgl[])
                  }
                  frame Error {
                    n113 = call <vilib>:"Clear Errors.vi"("error in (no error)"=w363, "specific error code to clear (0: all)"=43) -> ("error out"=w362:errorcluster)  [unwired: 4 in, 1 out]
                    n114 = for {
                      N: 64 -> [_]
                      tunnel: [0] -> w364 mode=indexing
                    }
                  }
                }
                n115 = call "PhaseSet.vi"("相位输入"=w355, "HIFU"=TRUE, "error in (no error)"=w354, "chn num"="totle chnnum", "SeqNum"=w347, "connection ID in"=w349) -> ("error out"=w353:errorcluster, "SeqOUT"=w346:u32)  [unwired: 2 out]
              }
              frame True {
              }
            }
          }
        }
      }
      event "SETVOLT": Value Change {
        n116 = event-data() -> ("NewVal"=w374:bool)  [unwired: 1 in, 5 out]
        n117 = case shown="True" w376 {
          tunnel: w377 -> [w381 w386]
          tunnel: [w381 w387] -> w375
          tunnel: w374 -> [_ w385]
          tunnel: w373 -> [_ w384]
          tunnel: w372 -> [w379 w383]
          tunnel: [w379 w382] -> w371
          frame False {
            n118 = One Button Dialog(message="i2c connected failed") -> ()  [unwired: 1 in, 1 out]
          }
          frame True {
            n119 = case shown="False" w385 {
              tunnel: [w395 w410] -> w387
              tunnel: w386 -> [w394 w410]
              tunnel: w384 -> [w392 _]
              tunnel: w383 -> [w390 w409]
              tunnel: [w389 w409] -> w382
              frame False {
                n120 = call "File Dialog2"("error in"=w394) -> ("selected path"=w398:path, "error out"=w393:errorcluster)  [unwired: 11 in, 2 out]
                n121 = case shown="No Error" w393 {
                  selector: w393 -> [w399 w405]
                  tunnel: w398 -> [w402 _]
                  tunnel: [w401 w406] -> w397
                  tunnel: [w400 w404] -> w396
                  frame No Error {
                    n122 = call "readVoltFile.vi"("error in (no error)"=w399, "Path"=w402) -> ("error out"=w400:errorcluster, "Array"=w401:sgl[])
                  }
                  frame Error {
                    n123 = call <vilib>:"Clear Errors.vi"("error in (no error)"=w405, "specific error code to clear (0: all)"=43) -> ("error out"=w404:errorcluster)  [unwired: 4 in, 1 out]
                    n124 = for {
                      N: 64 -> [_]
                      tunnel: [0] -> w406 mode=indexing
                    }
                  }
                }
                n125 = property on="totle chnnum" class="DigNum (strict)"() -> ("Value"=w388:i16)  [unwired: 2 in, 2 out]
                n126 = call "VoltChnSet.vi"("电压输入"=w397, "HIFU"=TRUE, "error in (no error)"=w396, "chn num"=w388, "SeqNum"=w390, "connection ID in"=w392) -> ("error out"=w395:errorcluster, "SeqOUT"=w389:u32)  [unwired: 2 out]
              }
              frame True {
              }
            }
          }
        }
      }
      event "Scan": Value Change {
        n127 = event-data() -> ("NewVal"=w417:bool)  [unwired: 1 in, 4 out]
        n128 = And(x=w428, y=w427) -> (x .and. y?=w425:bool)
        n129 = And(x=w425, y=w426) -> (x .and. y?=w424:bool)
        n130 = case shown="True" w424 {
          tunnel: w423 -> [_ w443]
          tunnel: w422 -> [w431 w442]
          tunnel: w421 -> [_ w441]
          tunnel: [w431 w440] -> w420
          tunnel: [w430 w433] -> w413
          tunnel: w419 -> [w430 w434]
          tunnel: w418 -> [_ w439]
          tunnel: w417 -> [_ w438]
          tunnel: w414 -> [_ w437]
          tunnel: w416 -> [w429 w436]
          tunnel: [w429 w435] -> w415
          tunnel: w412 -> [_ w432]
          frame False {
          }
          frame True {
            n131 = case shown="False" w438 {
              tunnel: w443 -> [w455 _]
              tunnel: w442 -> [w454 w647]
              tunnel: w441 -> [w453 _]
              tunnel: [w446 w647] -> w440
              tunnel: w439 -> [w452 _]
              tunnel: w437 -> [w451 _]
              tunnel: w436 -> [w449 w646]
              tunnel: [w450 w646] -> w435
              tunnel: w434 -> [_ w645]
              tunnel: [w445 w645] -> w433
              tunnel: w432 -> [w444 _]
              frame False {
                # "Scan path"
                # "osc"
                # "KYCT"
                n132 = property on="Position" class="Arr (strict)"() -> ("Value"=w456:dbl[])  [unwired: 2 in, 2 out]
                n133 = stacked-sequence {
                  seq-local: [w459 _ _] -> [_ w531 w629]
                  seq-local: [w463 _ _] -> [_ w529 _]
                  seq-local: [w462 _ _] -> [_ w536 _]
                  seq-local: [w461 _ _] -> [_ w528 _]
                  seq-local: [w457 _ _] -> [_ w530 w628]
                  seq-local: [_ w526 _] -> [_ _ w633]
                  seq-local: [w458 _ _] -> [_ w524 w625]
                  tunnel: w456 -> [w467 w523 _]
                  tunnel: w455 -> [_ w535 w622]
                  tunnel: w454 -> [w465 _ _]
                  tunnel: w453 -> [_ w534 _]
                  tunnel: [_ w527 _] -> w446
                  tunnel: w452 -> [_ _ _]
                  tunnel: w451 -> [_ w532 _]
                  tunnel: w449 -> [_ w533 _]
                  tunnel: [_ w525 _] -> w450
                  tunnel: "KYCT coordinate" -> [w460 _ _]
                  tunnel: "KYCT axis in HIFU coordinate" -> [w468 _ _]
                  tunnel: [_ _ w621] -> w445
                  tunnel: w444 -> [_ _ w624]
                  frame #0 {
                    # "Creat Scan Path"
                    n134 = Current VI's Path() -> (path=w466:path)
                    n135 = call "File Dialog"("start path"=w466, "error in"=w465) -> ("selected path"=w463:path, "error out"=w464:errorcluster)  [unwired: 10 in, 2 out]
                    n136 = call "ScanPath.vi"("Scan parameters"=w460, "Axis parameters"=w468, "Position"=w467, "error in (no error)"=w464) -> ("Scanmode"=w459:enum16{"X", "Y", "Z", "YZ", "XZ", "XY"}, "ScanPath"=w462:T5, "Scan Ready"=w458:bool, "Ticks"=w457:dbl[][], "error out"=w461:errorcluster)
                    n137 = case shown="\"XZ\"" w459 {
                      tunnel: w460 -> [w474 w480 w486 w498 w510 w522]
                      frame "X" {
                        n138 = Unbundle By Name(w474) -> ("X step"=w470:dbl, "X+"=w469:dbl, "X-"=w471:dbl)
                        n139 = property on="1D plot" class="XYGraph (strict)"("XScale.Increment"=w470, "XScale.Maximum"=w469, "XScale.Minimum"=w471, "XScale.MinorInc"=w470, "XScale.RngStart"=w471, "XScale.NameLbl.Text"="X" ("X Scale.Name Label.Text")) -> ()  [unwired: 2 in, 2 out]
                        n140 = local write "Tab Control"(enum32{"1D Scan", "2D Scan", "Monitor"}."1D Scan" ("Tab Control")) -> ()
                      }
                      frame "Y" {
                        n141 = Unbundle By Name(w480) -> ("Y step"=w476:dbl, "Y+"=w475:dbl, "Y-"=w477:dbl)
                        n142 = property on="1D plot" class="XYGraph (strict)"("XScale.Increment"=w476, "XScale.Maximum"=w475, "XScale.Minimum"=w477, "XScale.MinorInc"=w476, "XScale.RngStart"=w477, "XScale.NameLbl.Text"="X" ("X Scale.Name Label.Text")) -> ()  [unwired: 2 in, 2 out]
                        n143 = local write "Tab Control"(enum32{"1D Scan", "2D Scan", "Monitor"}."1D Scan" ("Tab Control")) -> ()
                      }
                      frame "Z" {
                        n144 = Unbundle By Name(w486) -> ("Z step"=w482:dbl, "Z+"=w481:dbl, "Z-"=w483:dbl)
                        n145 = property on="1D plot" class="XYGraph (strict)"("XScale.Increment"=w482, "XScale.Maximum"=w481, "XScale.Minimum"=w483, "XScale.MinorInc"=w482, "XScale.RngStart"=w483, "XScale.NameLbl.Text"="X" ("X Scale.Name Label.Text")) -> ()  [unwired: 2 in, 2 out]
                        n146 = local write "Tab Control"(enum32{"1D Scan", "2D Scan", "Monitor"}."1D Scan" ("Tab Control")) -> ()
                      }
                      frame "YZ" {
                        n147 = Unbundle By Name(w498) -> ("Y step"=w490:dbl, "Y+"=w492:dbl, "Y-"=w491:dbl, "Z step"=w487:dbl, "Z+"=w489:dbl, "Z-"=w488:dbl)
                        n148 = Add(x=w492, y=w491) -> (x+y=w497:dbl)
                        n149 = Add(x=w489, y=w488) -> (x+y=w496:dbl)
                        n150 = property on="2D Scan" class="IntGraph (strict)"("XScale.Multiplier"=w490, "XScale.Offset"=w497, "YScale.Multiplier"=w487, "YScale.Offset"=w496, "XScale.Increment"=w490, "XScale.Maximum"=w492, "XScale.Minimum"=w491, "YScale.Increment"=w487, "YScale.Maximum"=w489, "YScale.Minimum"=w488, "XScale.NameLbl.Text"="Z" ("X Scale.Name Label.Text"), "YScale.NameLbl.Text"="Y" ("Y Scale.Name Label.Text")) -> ()  [unwired: 2 in, 2 out]
                        n151 = local write "Tab Control"(enum32{"1D Scan", "2D Scan", "Monitor"}."2D Scan" ("Tab Control")) -> ()
                      }
                      frame "XZ" {
                        n152 = Unbundle By Name(w510) -> ("X step"=w502:dbl, "X+"=w504:dbl, "X-"=w503:dbl, "Z step"=w499:dbl, "Z+"=w501:dbl, "Z-"=w500:dbl)
                        n153 = Add(x=w504, y=w503) -> (x+y=w509:dbl)
                        n154 = Add(x=w501, y=w500) -> (x+y=w508:dbl)
                        n155 = property on="2D Scan" class="IntGraph (strict)"("YScale.Multiplier"=w502, "YScale.Offset"=w509, "XScale.Multiplier"=w499, "XScale.Offset"=w508, "YScale.Increment"=w502, "YScale.Maximum"=w504, "YScale.Minimum"=w503, "XScale.Increment"=w499, "XScale.Maximum"=w501, "XScale.Minimum"=w500, "YScale.NameLbl.Text"="Z" ("X Scale.Name Label.Text"), "XScale.NameLbl.Text"="X" ("Y Scale.Name Label.Text")) -> ()  [unwired: 2 in, 2 out]
                        n156 = local write "Tab Control"(enum32{"1D Scan", "2D Scan", "Monitor"}."2D Scan" ("Tab Control")) -> ()
                      }
                      frame "XY" {
                        n157 = Unbundle By Name(w522) -> ("X step"=w514:dbl, "X+"=w516:dbl, "X-"=w515:dbl, "Y step"=w511:dbl, "Y+"=w513:dbl, "Y-"=w512:dbl)
                        n158 = Add(x=w516, y=w515) -> (x+y=w521:dbl)
                        n159 = Add(x=w513, y=w512) -> (x+y=w520:dbl)
                        n160 = property on="2D Scan" class="IntGraph (strict)"("YScale.Multiplier"=w514, "YScale.Offset"=w521, "XScale.Multiplier"=w511, "XScale.Offset"=w520, "YScale.Increment"=w514, "YScale.Maximum"=w516, "YScale.Minimum"=w515, "XScale.Increment"=w511, "XScale.Maximum"=w513, "XScale.Minimum"=w512, "YScale.NameLbl.Text"="Y" ("X Scale.Name Label.Text"), "XScale.NameLbl.Text"="X" ("Y Scale.Name Label.Text")) -> ()  [unwired: 2 in, 2 out]
                        n161 = local write "Tab Control"(enum32{"1D Scan", "2D Scan", "Monitor"}."2D Scan" ("Tab Control")) -> ()
                      }
                    }
                  }
                  frame #1 {
                    # "Scan"
                    n162 = case shown="True" w524 {
                      tunnel: w536 -> [_ w558]
                      tunnel: w535 -> [_ w557]
                      tunnel: w534 -> [_ w556]
                      tunnel: w533 -> [w540 w555]
                      tunnel: w532 -> [_ w554]
                      tunnel: w531 -> [_ w553]
                      tunnel: w530 -> [_ w551]
                      tunnel: w529 -> [_ w549]
                      tunnel: w528 -> [w539 w548]
                      tunnel: [w539 w546] -> w527
                      tunnel: [dbl[][] [] w545] -> w526
                      tunnel: [w540 w544] -> w525
                      tunnel: [w537 w543] -> _
                      tunnel: w523 -> [w537 _]
                      frame False {
                        # "wrong scan dimension"
                      }
                      frame True {
                        n163 = while {
                          tunnel: w558 -> [w568]
                          tunnel: w557 -> [w601]
                          tunnel: w556 -> [w599]
                          tunnel: w554 -> [w593]
                          shift-right: [w592] -> w544
                          shift-left: w555 -> [w596]
                          tunnel: w549 -> [w583]
                          tunnel: [w577] -> w545 mode=indexing
                          tunnel: w553 -> [w576]
                          shift-right: [w571] -> _
                          shift-left: dbl[] [] -> [w574]
                          tunnel: w551 -> [w572]
                          shift-right: [w570] -> w547
                          shift-left: w548 -> [w603]
                          tunnel: [w561] -> w543
                          i -> [w565]
                          stop <- w562 stop-if-true
                          n164 = property on="cycle" class="DigNum (strict)"() -> ("Value"=w598:u32)  [unwired: 2 in, 2 out]
                          n165 = property on="record cycle" class="DigNum (strict)"() -> ("Value"=w560:u64)  [unwired: 2 in, 2 out]
                          n166 = Index Array(array=w568, index (row)=w565) -> (element=w602:dbl[])  [unwired: 1 in]
                          n167 = property on="freq (MHz)" class="DigNum (strict)"() -> ("Value"=w559:dbl)  [unwired: 2 in, 2 out]
                          n168 = Array Size(array=w568) -> (size(s)=w567:i32[])
                          n169 = Greater?(x=w576, y=enum16{"X", "Y", "Z", "YZ", "XZ", "XY"}."Z" ("Scanmode")) -> (0:w575:bool)
                          n170 = Increment(x=w565) -> (x+1=w563:i32)
                          n171 = Index Array(array=w567, index=0) -> (element=w564:i32)
                          n172 = property on="Position" class="Arr (strict)"() -> ("Value"=w600:dbl[])  [unwired: 2 in, 2 out]
                          n173 = property on="Channel" class="DigNum (strict)"() -> ("Value"=w595:u16)  [unwired: 2 in, 2 out]
                          n174 = Less Or Equal?(x=w564, y=w563) -> (x <= y?=w562:bool)
                          n175 = call "move.vi"("error in (no error)"=w603, "P01"=w602, "P0"=w600, "UART PORT in"=w601) -> ("error out"=w594:errorcluster, "P1"=w561:dbl[])  [unwired: 1 out]
                          n176 = call "pulsedRead.vi"("osc in"=w599, "connection ID"=w593, "recCycles"=w560, "channel"=w595, "error in (no error)"=w594, "freq (MHz)"=w559, "cycles"=w598, "points"=u64 8000, "SEQ IN"=w596) -> ("error out"=w590:errorcluster, "voltage"=w579:dbl[], "SEQ OUT"=w592:u32, "time"=w580:dbl[])  [unwired: 1 in, 2 out]
                          n177 = property on="Position" class="Arr (strict)"("Value"=w561) -> ()  [unwired: 2 in, 2 out]
                          n178 = Number To Decimal String(number=w565) -> (decimal integer string=w588:string)  [unwired: 1 in]
                          n179 = Build Array(w580, w579) -> (w591:T5)
                          n180 = Concatenate Strings("POINT" ("string"), w588, ".txt" ("string")) -> (w585:string)
                          n181 = Build Path(base path=w583, name or relative path=w585) -> (appended path=w584:path)
                          n182 = call-poly <vilib>:"Write Delimited Spreadsheet.vi"("file path (dialog if empty)"=w584, "format (%.3f)"="%.8e", "2D data"=w591, "error in (no error)"=w590) -> ("error out"=w578:errorcluster)  [unwired: 10 in, 1 out]
                          n183 = Bundle("time"=w580, "voltage"=w579) -> (w582:cluster{"time":dbl[], "voltage":dbl[]})  [unwired: 1 in]
                          n184 = property on="Sens (V/MPa)" class="DigNum (strict)"() -> ("Value"=w581:dbl)  [unwired: 2 in, 2 out]
                          n185 = property on="XY Graph 2" class="XYGraph (strict)"("Value"=w582) -> ()  [unwired: 2 in, 2 out]
                          n186 = call "findMag.vi"("times"=w580, "sens"=w581, "voltages"=w579, "error in (no error)"=w578, "freq"=w559) -> ("magfound"=w573:dbl, "error out"=w570:errorcluster)
                          n187 = Build Array (concatenate)(w561, w573) -> (w577:dbl[])
                          n188 = Build Array (concatenate)(w574, w573) -> (w571:dbl[])
                          n189 = case shown="True" w575 {
                            tunnel: w572 -> [w611 w618]
                            tunnel: w571 -> [w610 w620]
                            frame False {
                              w609 = 0 ("index")
                              # "1D plot"
                              n190 = Array Size(array=w610) -> (size(s)=w606:i32)
                              n191 = Array Subset(array=w611, index (row)=w609, length (row)=1 ("length"), index (col)=w609, length (col)=w606) -> (w607:dbl[][])
                              n192 = Reshape Array(w607, w606) -> (w605:dbl[])
                              n193 = Bundle(w605, w610) -> (w604:cluster{dbl[], dbl[]})  [unwired: 1 in]
                              n194 = property on="1D plot" class="XYGraph (strict)"("Value"=w604) -> ()  [unwired: 2 in, 2 out]
                            }
                            frame True {
                              # "2D Scan"
                              n195 = Index Array(array=w618, index (row) #1=1 ("index (row)"), index (col) #1=3 ("disabled index (col)"), index (row) #2=0 ("index (row)"), index (col) #2=3 ("disabled index (col)")) -> (element #1=w613:dbl, element #2=w612:dbl)
                              n196 = Reshape Array(w620, w613, w612) -> (w619:dbl[][])
                              n197 = property on="2D Scan" class="IntGraph (strict)"("Value"=w619) -> ()  [unwired: 2 in, 2 out]
                            }
                          }
                          n198 = property on="Pressure (MPa)" class="DigNum (strict)"("Value"=w573) -> ()  [unwired: 2 in, 2 out]
                        }
                        n199 = Build Path(base path=w549, name or relative path="Data.txt") -> (appended path=w542:path)
                        n200 = call-poly <vilib>:"Write Delimited Spreadsheet.vi"("file path (dialog if empty)"=w542, "format (%.3f)"="%.3f", "2D data"=w545, "error in (no error)"=w547) -> ("error out"=w546:errorcluster)  [unwired: 10 in, 1 out]
                      }
                    }
                  }
                  frame #2 {
                    # "matlab display"
                    n201 = property on="Position" class="Arr (strict)"() -> ("Value"=w623:dbl[])  [unwired: 2 in, 2 out]
                    n202 = call "move.vi"("P01"=w624, "P0"=w623, "UART PORT in"=w622) -> ("P1"=w621:dbl[])  [unwired: 1 in, 2 out]
                    n203 = property on="Position" class="Arr (strict)"("Value"=w621) -> ()  [unwired: 2 in, 2 out]
                    n204 = Two Button Dialog(message="Create MATLAB figure?", 1:"NO" ("F button name (\"Cancel\")"), 2:"YES" ("T button name (\"OK\")")) -> (T button?=w627:bool)
                    n205 = And(x=w625, y=w627) -> (x .and. y?=w626:bool)
                    n206 = case shown="True" w626 {
                      tunnel: w633 -> [_ w638]
                      tunnel: w629 -> [_ w636]
                      tunnel: w628 -> [_ w634]
                      frame False {
                      }
                      frame True {
                        n207 = Greater?(x=w636, y=enum16{"X", "Y", "Z", "YZ", "XZ", "XY"}."Z" ("Scanmode")) -> (0:w637:bool)
                        n208 = case shown="True" w637 {
                          tunnel: w638 -> [w641 w644]
                          tunnel: w636 -> [w640 w642]
                          tunnel: w634 -> [w639 w643]
                          frame False {
                            # "1D Scan"
                            n209 = script code="% data=load('Data1.txt');\n% Ticks = [-20:0.5:20;-20:0.5:20];\n% ScanMode = 0;\n%% begin\nglobal data Ticks ScanMode\nfig = figure;\nresizefactor = 4;\nxvec = data(:,1);\nyvec = data(:,2);\nzvec = data(:,3);\nPvec = data(:,4);\nHIFUxvec = Ticks(1,:);\nh1 = plot(HIFUxvec,Pvec);\ndcm_obj = datacursormode(fig);\nset(dcm_obj,'UpdateFcn',@cursorfunc); \nswitch ScanMode\n    case 0\n        labelx = 'X in HIFU Coord (mm)';\n    case 1\n        labelx = 'Y in HIFU Coord (mm)';\n    case 2\n        labelx = 'Z in HIFU Coord (mm)';\nend\nxlabel(labelx);\nylabel('Acousctic pressure (MPa)');"("data"=w641, "ScanMode"=w640, "Ticks"=w639) -> ()  [unwired: 1 in, 1 out]
                          }
                          frame True {
                            # "2D Scan"
                            n210 = script code="% data=load('Data2.txt');\n% Ticks = [-15,1,15,31;-8,0.5,8,33];\n% ScanMode = 5;\n%% begin\nglobal data Ticks ScanMode\nfig = figure;\nresizefactor = 4;\nxvec = data(:,1);\nyvec = data(:,2);\nzvec = data(:,3);\nPvec = data(:,4);\nHIFUxvec = Ticks(1,1):Ticks(1,2):Ticks(1,3);\nHIFUyvec = Ticks(2,1):Ticks(2,2):Ticks(2,3);\nHIFUxnum = Ticks(1,4);\nHIFUynum = Ticks(2,4);\nPmap = reshape(Pvec,HIFUxnum,HIFUynum);%反过来\nh1 = imagesc(HIFUyvec,HIFUxvec,Pmap);%反过来\ndcm_obj = datacursormode(fig);\nset(dcm_obj,'UpdateFcn',@cursorfunc); \nswitch ScanMode\n    case 3\n        labely = 'Y in HIFU Coord (mm)';\n        labelx = 'Z in HIFU Coord (mm)';\n    case 4\n        labely = 'X in HIFU Coord (mm)';\n        labelx = 'Z in HIFU Coord (mm)';\n    case 5\n        labely = 'X in HIFU Coord (mm)';\n        labelx = 'Y in HIFU Coord (mm)';\nend\nxlabel(labelx);\nylabel(labely);\ncolormap('jet');\nhcb = colorbar;\nylabel(hcb,'Acousctic pressure (MPa)')"("data"=w644, "Ticks"=w643, "ScanMode"=w642) -> ()  [unwired: 1 in, 1 out]
                          }
                        }
                      }
                    }
                  }
                }
              }
              frame True {
              }
            }
          }
        }
      }
      event "pout": Value Change {
        n211 = event-data() -> ("NewVal"=w653:bool)  [unwired: 1 in, 5 out]
        n212 = And(x=w656, y=w655) -> (x .and. y?=w654:bool)
        n213 = case shown="False" w653 {
          tunnel: w659 -> [w667 _]
          tunnel: w658 -> [w666 w688]
          tunnel: [w665 w688] -> w657
          tunnel: w654 -> [w664 _]
          tunnel: w652 -> [w663 w687]
          tunnel: w650 -> [w662 _]
          tunnel: [w661 w687] -> w651
          frame False {
            n214 = case shown="True" w664 {
              tunnel: w667 -> [_ w686]
              tunnel: w666 -> [w670 w685]
              tunnel: [w670 w680] -> w665
              tunnel: w663 -> [w668 w679]
              tunnel: w662 -> [_ w678]
              tunnel: [w668 w677] -> w661
              frame False {
                n215 = One Button Dialog(message="HIFU或示波器没有连接！") -> ()  [unwired: 1 in, 1 out]
              }
              frame True {
                n216 = property on="record cycle" class="DigNum (strict)"() -> ("Value"=w672:u64)  [unwired: 2 in, 2 out]
                n217 = property on="freq (MHz)" class="DigNum (strict)"() -> ("Value"=w671:dbl)  [unwired: 2 in, 2 out]
                n218 = property on="Channel" class="DigNum (strict)"() -> ("Value"=w673:u16)  [unwired: 2 in, 2 out]
                n219 = property on="cycle" class="DigNum (strict)"() -> ("Value"=w674:u32)  [unwired: 2 in, 2 out]
                n220 = call "pulsedRead.vi"("osc in"=w686, "connection ID"=w678, "recCycles"=w672, "channel"=w673, "error in (no error)"=w685, "freq (MHz)"=w671, "cycles"=w674, "points"=u64 20000, "SEQ IN"=w679) -> ("error out"=w681:errorcluster, "voltage"=w682:dbl[], "SEQ OUT"=w677:u32, "time"=w683:dbl[])  [unwired: 1 in, 2 out]
                n221 = property on="pulsedRead.viSens (V/MPa)" class="DigNum (strict)"() -> ("Value"=w676:dbl)  [unwired: 2 in, 2 out]
                n222 = call "findMag.vi"("times"=w683, "sens"=w676, "voltages"=w682, "error in (no error)"=w681, "freq"=w671) -> ("magfound"=w675:dbl, "error out"=w680:errorcluster)
                n223 = property on="Pressure (MPa)" class="DigNum (strict)"("Value"=w675) -> ()  [unwired: 2 in, 2 out]
              }
            }
          }
          frame True {
          }
        }
      }
      event "oscilloscope": Value Change {
        # "Osc initiation"
        n224 = event-data() -> ()  [unwired: 1 in, 6 out]
        n225 = VISA Open(error in (no error)=w699, VISA resource name="oscilloscope") -> (VISA resource name=w690:refnum<visa-resource-name>, error out=w692:errorcluster)  [unwired: 3 in]
        n226 = VISA Write(VISA resource name=w690, write buffer=":ACQuire:TYPE HRESolution", error in (no error)=w692) -> (error out=w691:errorcluster)  [unwired: 2 out]
        n227 = property on="osc" class="Bool (strict)"(error in=w691, "Value"=TRUE) -> (error out=w698:errorcluster)  [unwired: 1 in, 1 out]
      }
      event "HIFU_connect": Value Change {
        n228 = event-data() -> ("NewVal"=w708:bool)  [unwired: 1 in, 5 out]
        n229 = case shown="False" w708 {
          tunnel: w709 -> [w712 w741]
          tunnel: [w717 w741] -> w707
          tunnel: [w716 FALSE] -> w706
          tunnel: [w714 refnum<k5> refnum ("connection ID")] -> w705
          tunnel: [w713 u32 0] -> w704
          frame False {
            n230 = call <vilib>:"Simple Error Handler.vi"("error in (no error)"=w712) -> ("error out"=w711:errorcluster)  [unwired: 4 in, 4 out]
            n231 = TCP Open Connection(address="HIFU IP", remote port or service name="Port", timeout ms (60000)=10000, error in (no error)=w711) -> (connection ID=w715:refnum<k5>, error out=w718:errorcluster)  [unwired: 1 in]
            n232 = case shown="No Error" w718 {
              selector: w718 -> [w725 w735]
              tunnel: [w723 w734] -> w717
              tunnel: [TRUE FALSE] -> w716
              tunnel: w715 -> [w727 _]
              tunnel: [w724 refnum<k5> refnum ("connection ID")] -> w714
              tunnel: [u32 0 u32 0] -> w713
              frame No Error {
                n233 = property on="freq (MHz)" class="DigNum (strict)"() -> ("Value"=w722:dbl)  [unwired: 2 in, 2 out]
                n234 = call "freqSet.vi"("error in (no error)"=w725, "SEQ in"=u32 0, "freq(MHz)"=w722, "connection ID"=w727) -> ("error out"=w723:errorcluster, "connection ID out"=w724:refnum<k5>)  [unwired: 2 out]
              }
              frame Error {
                # "Timeout"
                n235 = Unbundle By Name(w735) -> ("code"=w736:i32)
                n236 = case shown="56" w736 {
                  tunnel: w735 -> [w737 _]
                  tunnel: [w737 w738] -> w734
                  frame Default {
                  }
                  frame 56 {
                    w738 = errorcluster {"status"=FALSE, "code"=0, "source"=""}  # No error
                  }
                }
                n237 = One Button Dialog(message="Connecting HIFU failed. Timeout.") -> ()  [unwired: 1 in, 1 out]
              }
            }
          }
          frame True {
          }
        }
        n238 = property on="HIFU" class="Bool (strict)"("Value"=w706) -> ()  [unwired: 2 in, 2 out]
      }
      event "freq (MHz)": Value Change {
        n239 = event-data() -> ()  [unwired: 1 in, 6 out]
      }
      event "Set global voltage": Value Change {
        n240 = event-data() -> ("NewVal"=w755:bool)  [unwired: 1 in, 5 out]
        n241 = case shown="False" w755 {
          tunnel: w760 -> [w767 w780]
          tunnel: [w766 w780] -> w759
          tunnel: w758 -> [w765 _]
          tunnel: w756 -> [w764 _]
          tunnel: w752 -> [w763 _]
          tunnel: w754 -> [w762 w779]
          tunnel: [w761 w779] -> w753
          frame False {
            n242 = case shown="True" w764 {
              tunnel: w767 -> [w769 w777]
              tunnel: [w769 w776] -> w766
              tunnel: w765 -> [_ w775]
              tunnel: w763 -> [_ w773]
              tunnel: w762 -> [w768 w772]
              tunnel: [w768 w771] -> w761
              frame False {
                n243 = One Button Dialog(message="i2c AMP connecting failed") -> ()  [unwired: 1 in, 1 out]
              }
              frame True {
                n244 = call "voltageSet.vi"("error in (no error)"=w777, "SEQ in"=w772, "Voltage"=w775, "connection ID"=w773) -> ("error out"=w776:errorcluster, "SEQ out"=w771:u32, "OK？"=w774:bool)  [unwired: 1 out]
                n245 = case shown="False" w774 {
                  frame True {
                  }
                  frame False {
                    n246 = One Button Dialog(message="Seting voltage failed") -> ()  [unwired: 1 in, 1 out]
                  }
                }
              }
            }
          }
          frame True {
          }
        }
      }
      event "continuousOut": Value Change {
        n247 = event-data() -> ()  [unwired: 1 in, 6 out]
        n248 = case shown="False" w796 {
          tunnel: w795 -> [_ w835]
          tunnel: [_ w835] -> w794
          frame False {
          }
          frame True {
          }
        }
        n249 = case shown="False" "continuousOut" {
          tunnel: [0 1] -> w793
          tunnel: [FALSE TRUE] -> _
          frame False {
          }
          frame True {
          }
        }
        n250 = case shown="True" w789 {
          tunnel: w793 -> [_ w801]
          tunnel: w792 -> [w799 w805]
          tunnel: [w799 w804] -> w791
          tunnel: w788 -> [_ _]
          tunnel: w787 -> [w797 w807]
          tunnel: w786 -> [w798 w806]
          tunnel: [w798 w803] -> w785
          tunnel: [w797 w802] -> w784
          frame False {
          }
          frame True {
            n251 = case shown="1" w801 {
              tunnel: w807 -> [w813 w828]
              tunnel: w806 -> [w814 w827]
              tunnel: w805 -> [_ w825]
              tunnel: [w810 w824] -> w804
              tunnel: [w811 w822] -> w803
              tunnel: [w812 w821] -> w802
              tunnel: [w808 w818] -> w800
              frame 0, Default {
                n252 = call "STOPheat.vi"("connection ID"=w813, "SEQ in"=w814) -> ("connection ID out"=w812:refnum<k5>, "SEQ out"=w811:u32, "OK?"=w809:bool, "error out"=w810:errorcluster)  [unwired: 1 in]
                n253 = case shown="True" w809 {
                  tunnel: [w815 FALSE] -> w808
                  frame False {
                    n254 = property on="Sonication" class="Bool (strict)"() -> ("Value"=w815:bool)  [unwired: 2 in, 2 out]
                  }
                  frame True {
                  }
                }
              }
              frame 1 {
                n255 = property on="totle chnnum" class="DigNum (strict)"() -> ("Value"=w826:i16)  [unwired: 2 in, 2 out]
                n256 = property on="Channel" class="DigNum (strict)"() -> ("Value"=w817:u16)  [unwired: 2 in, 2 out]
                n257 = call "PulsedOut.vi"("Cycles"=u64 360000000000000, "Channel"=w817, "frequency (MHz)"=1.367, "error in (no error)"=w825, "SEQ IN"=w827, "chn num"=w826, "connection ID"=w828) -> ("error out"=w824:errorcluster, "OK?"=w819:bool, "connection ID out"=w821:refnum<k5>, "SEQ OUT"=w822:u32)
                n258 = case shown="False" w819 {
                  tunnel: [w829 TRUE] -> w818
                  frame False {
                    n259 = property on="Sonication" class="Bool (strict)"() -> ("Value"=w829:bool)  [unwired: 2 in, 2 out]
                  }
                  frame True {
                  }
                }
              }
            }
            "Sonication" <- w800
          }
        }
      }
    }
    n260 = case shown="True" "HIFU_Telnet" {
      tunnel: w18 -> [_ w37]
      frame False {
      }
      frame True {
        n261 = stacked-sequence {
          tunnel: w37 -> [_ _ w41]
          frame #0 {
            n262 = property on="HIFU_Telnet" class="Bool (strict)"("DisabledEnum"=T3."Disabled" ("Disabled")) -> ()  [unwired: 2 in, 2 out]
          }
          frame #1 {
            n263 = property on="HIFU" class="Bool (strict)"("Value"=FALSE) -> ()  [unwired: 2 in, 2 out]
            n264 = property on="HIFU IP" class="Str"() -> ("Value"=w39:string)  [unwired: 2 in, 2 out]
            n265 = call "telnet_com.vi"("HIFU ip"=w39) -> ()
          }
          frame #2 {
            n266 = property on="HIFU" class="Bool (strict)"("Value"=w41) -> ()  [unwired: 2 in, 2 out]
            n267 = property on="HIFU_Telnet" class="Bool (strict)"("DisabledEnum"=T3."Enabled" ("Disabled"), "Value"=FALSE ("HIFU_Telnet")) -> ()  [unwired: 2 in, 2 out]
          }
        }
      }
    }
    n268 = property on="Position" class="Arr (strict)"("Value"=w34) -> ()  [unwired: 2 in, 2 out]
    "Current" <- w16
    "Voltage" <- w10
    "error out" <- w20
  }
